vi "Get Clock.vi"(0 "Ethernet MAC - Custom.lvclass":refnum<class "Ethernet MAC - Custom.lvclass">) -> (8 "MAC Clock":refnum<k21>)   [LabVIEW 2020, in "Ethernet MAC - Custom.lvclass"]
uses:
  Ethernet MAC - Custom.lvclass
  <instrlib>/_niInstr/Network/Ethernet/MAC/API/v1/FPGA/niInstr Ethernet MAC v1.lvclass
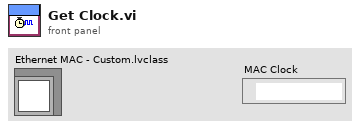
[diagram p1: front panel]
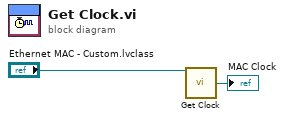
[diagram p0: block diagram]
diagram:
  n1 = call-parent "Get Clock.vi"("niInstr Ethernet MAC v1.lvclass"="Ethernet MAC - Custom.lvclass") -> ("MAC Clock"=→"MAC Clock":refnum<k21>)  [unwired: 14 in]
